vi "Test_1.vi"() -> ()   [LabVIEW 2017]
uses:
  <vilib>/Utility/file.llb/Read From Spreadsheet File (I64).vi
panel:
  out "XY Graph":cluster{i64[], i64[]}(graph)
  in  "file path X":path=path "c:/test.txt"
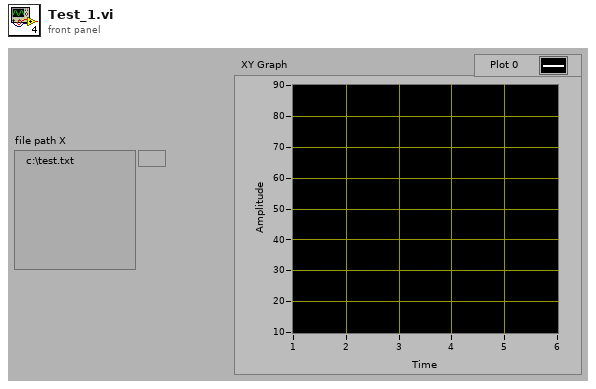
[diagram p1: front panel]
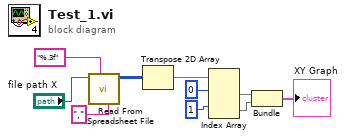
[diagram p0: block diagram]
diagram:
  n1 = call-poly <vilib>:"Read From Spreadsheet File.vi"("delimiter (\\t)"="," ("delimiter (\\t)"), "format (%d)"="%.3f" ("format (%.3f)"), "file path (dialog if empty)"="file path X") -> ("all rows"=w3:i64[][])  [unwired: 4 in, 4 out]
  n2 = Transpose 2D Array(2D array=w3) -> (transposed array=w2:i64[][])
  n3 = Index Array(array=w2, index (row) #1=0 ("index (row)"), index (row) #2=1 ("index (row)")) -> (element #1=w6:i64[], element #2=w5:i64[])  [unwired: 2 in]
  n4 = Bundle(w6, w5) -> (→"XY Graph":cluster{i64[], i64[]})  [unwired: 1 in]
